vi "Read ProtocolConfig.vi"(8 "error in (no error)":errorcluster, 11 "FTPProtocol in":refnum<class "FTPProtocol.lvclass">) -> (0 "error out":errorcluster, 2 "ProtocolConfig.lvclass":refnum<class "ProtocolConfig.lvclass">, 3 "FTPProtocol out":refnum<class "FTPProtocol.lvclass">)   [LabVIEW 2014, in "FileSync -- FTP.lvlib" / "FTPProtocol.lvclass"]
uses:
  FTPProtocol.lvclass
  Base/ProtocolConfig/ProtocolConfig.lvclass
  FTPProtocol.lvclass/FTPProtocol.ctl
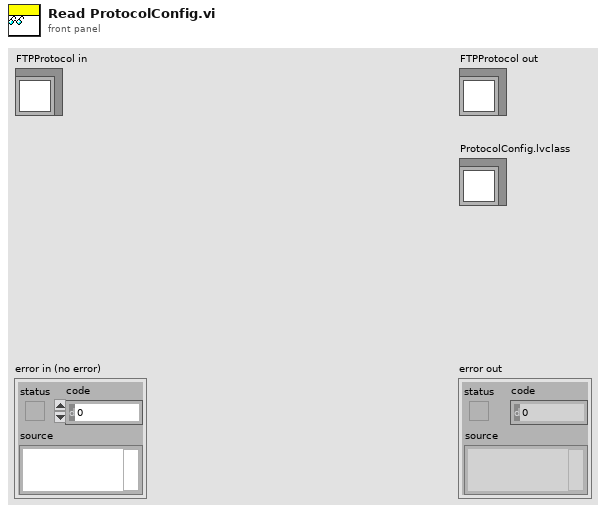
[diagram p1: front panel]
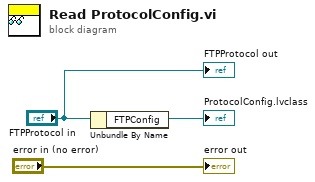
[diagram p0: block diagram]
diagram:
  n1 = Unbundle By Name("FTPProtocol in") -> ("FTPConfig"=→"ProtocolConfig.lvclass":refnum<class "FTPConfig.lvclass">)
  "error out" <- "error in (no error)"
  "FTPProtocol out" <- "FTPProtocol in"
